vi "TwGetBufWriteProfileFromH5.vi"(0 "filename":string, 1 "profile in":sgl[](array[numeric]), 2 "peakIndex":i32, 3 "bufIndex":i32, 4 "error in (no error)":errorcluster) -> (5 "error out":errorcluster, 6 "profile out":sgl[](array[numeric]))   [LabVIEW 2009]
uses:
  TwH5Dll.dll
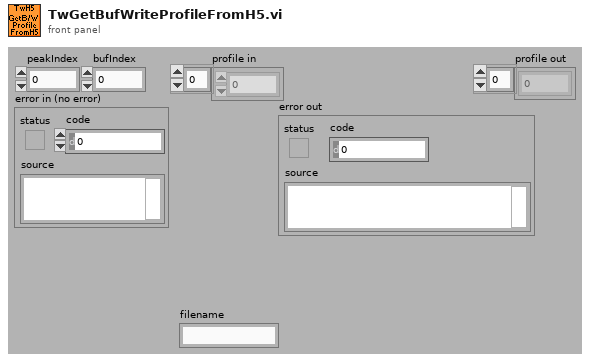
[diagram p1: front panel]
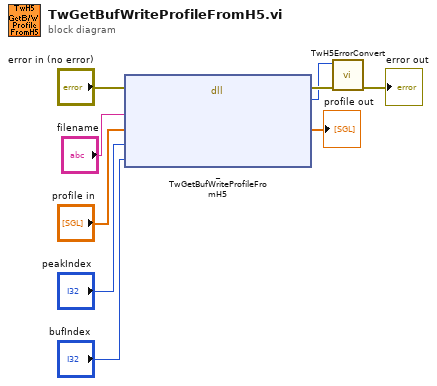
[diagram p0: block diagram]
diagram:
  n1 = dll-call lib="C:/src/85_TofDaq_current/DllWrappers/LabView/TwH5Dll/TwH5Dll.dll" fn="_TwGetBufWriteProfileFromH5"(error in="error in (no error)", "filename"="filename", "profile"="profile in", "peakIndex"="peakIndex", "segmentIndex"="bufIndex") -> (error out=w8:errorcluster, "TwRetVal"=w7:i32, "profile"=→"profile out":sgl[])  [unwired: 5 in, 1 out]
  n2 = call "TwH5ErrorConvert.vi"("error in (no error)"=w8, "error code"=w7) -> ("error out"=→"error out":errorcluster)  [unwired: 9 out]
